vi "conversion_Consigne_UI_Param_FPGA.vi"(10 "customParam":T1={"CamDelayToOpen(µs)"=10, "FLWidth(µs)"=10, "QSWidth(µs)"=10, "DelayFL_QS (µs)"=180, "CamDelayToClose(µs)"=100, "CamPivExposure(µs)"=100}, 11 "Config UI":T3) -> (3 "Config FPGA":T2 {"t_periode" min=1 max=999999 step=1})   [LabVIEW 2023]
uses:
  configUtilisateur.ctl
  configFPGA.ctl
  customParam.ctl
  modeAcq.ctl
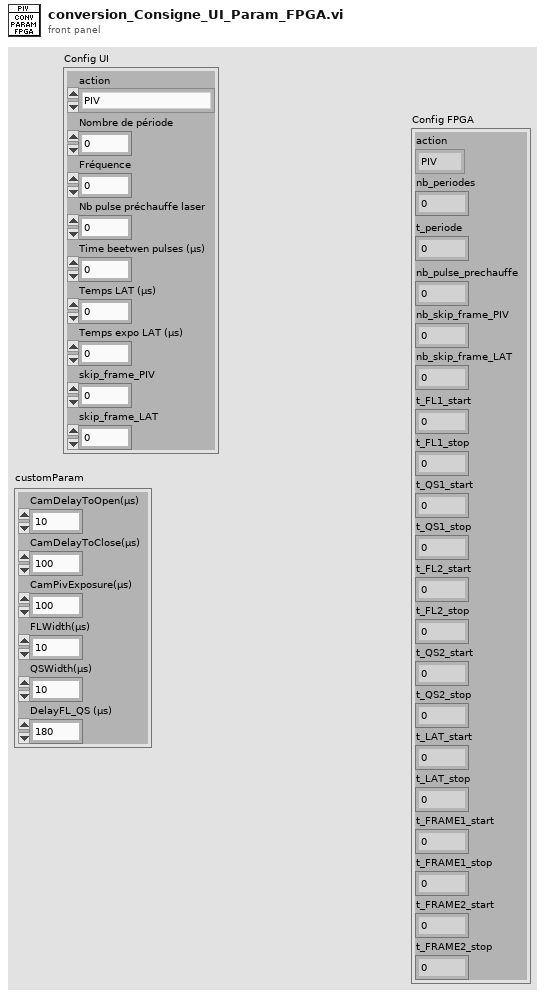
[diagram p1: front panel]
types:
  T1 = typedef "customParam.ctl" = cluster{"CamDelayToOpen(µs)":u32, "FLWidth(µs)":u32, "QSWidth(µs)":u32, "DelayFL_QS (µs)":u32, "CamDelayToClose(µs)":u32, "CamPivExposure(µs)":u32}
  T2 = typedef "configFPGA.ctl" = cluster{"action":enum8{"PIV", "PIV + LAT", "LAT", "STOP"}, "nb_periodes":u16, "t_periode":u32, "nb_pulse_prechauffe":u8, "nb_skip_frame_PIV":u8, "nb_skip_frame_LAT":u8, "t_FL1_start":u32, "t_FL1_stop":u32, "t_QS1_start":u32, "t_QS1_stop":u32, "t_FL2_start":u32, "t_FL2_stop":u32, "t_QS2_start":u32, "t_QS2_stop":u32, "t_LAT_start":u32, "t_LAT_stop":u32, "t_FRAME1_start":u32, "t_FRAME1_stop":u32, "t_FRAME2_start":u32, "t_FRAME2_stop":u32}
  T3 = typedef "configUtilisateur.ctl" = cluster{"Nombre de période":u16, "Fréquence ":u16, "Nb pulse préchauffe laser":u16, "skip_frame_PIV":u8, "skip_frame_LAT":u8, "Time beetwen pulses (µs)":u32, "Temps LAT (µs)":u32, "Temps expo LAT (µs)":u32, "action":enum8{"PIV", "PIV + LAT", "LAT"}}
  T4 = typedef "modeAcq.ctl" = enum8{"PIV", "PIV + LAT", "LAT", "STOP"}
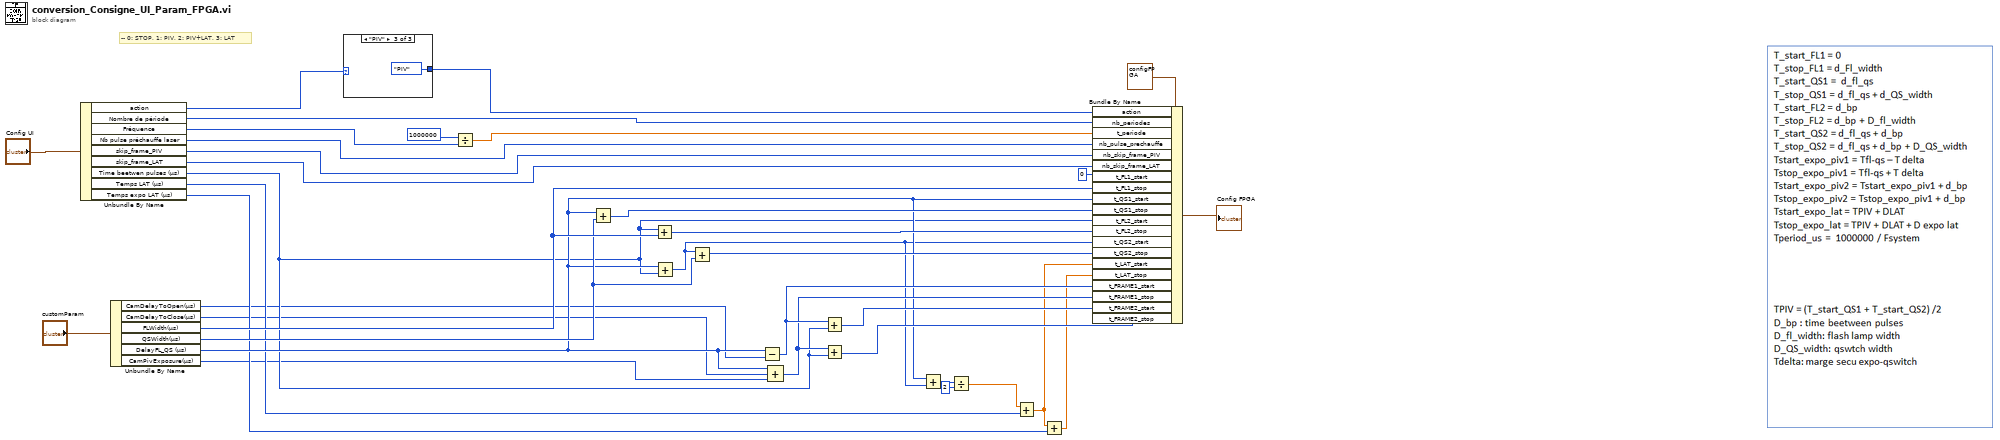
[diagram p0: block diagram]
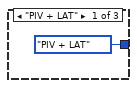
[diagram p2: hidden frame]
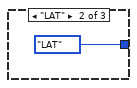
[diagram p3: hidden frame]
diagram:
  # "-- 0: STOP, 1: PIV, 2: PIV+LAT, 3: LAT"
  n1 = Unbundle By Name("Config UI") -> ("action"=w34:enum8{"PIV", "PIV + LAT", "LAT"}, "Nombre de période"=w33:u16, "Fréquence"=w31:u16, "Nb pulse préchauffe laser"=w29:u16, "skip_frame_PIV"=w28:u8, "skip_frame_LAT"=w27:u8, "Time beetwen pulses (µs)"=w12:u32, "Temps LAT (µs)"=w11:u32, "Temps expo LAT (µs)"=w10:u32)
  n2 = Unbundle By Name("customParam") -> ("CamDelayToOpen(µs)"=w4:u32, "CamDelayToClose(µs)"=w3:u32, "FLWidth(µs)"=w23:u32, "QSWidth(µs)"=w21:u32, "DelayFL_QS (µs)"=w16:u32, "CamPivExposure(µs)"=w2:u32)
  n3 = case shown="\"PIV\"" w34 {
    tunnel: [modeAcq."PIV + LAT" ("action") modeAcq."LAT" ("action") modeAcq."PIV" ("action")] -> w1
    frame "PIV + LAT" {
    }
    frame "LAT" {
    }
    frame "PIV" {
    }
  }
  n4 = Divide(x=1000000, y=w31) -> (x/y=w30:dbl)
  n5 = Add(x=w16, y=w21) -> (x+y=w25:u32)
  n6 = Add(x=w12, y=w23) -> (x+y=w24:u32)
  n7 = Add(x=w16, y=w12) -> (x+y=w15:u32)
  n8 = Add(x=w15, y=w21) -> (x+y=w22:u32)
  n9 = Subtract(x=w16, y=w4) -> (x-y=w20:u32)
  n10 = Compound Arithmetic op=ADD(w16, w3, w2) -> (w19:u32)
  n11 = Add(x=w20, y=w12) -> (x+y=w18:u32)
  n12 = Add(x=w19, y=w12) -> (x+y=w17:u32)
  n13 = Add(x=w16, y=w15) -> (x+y=w14:u32)
  n14 = Divide(x=w14, y=u32 2) -> (x/y=w7:dbl)
  n15 = Add(x=w7, y=w11) -> (x+y=w9:dbl)
  n16 = Add(x=w9, y=w10) -> (x+y=w8:dbl)
  n17 = Bundle By Name(cluster=T2 {"action"=enum."PIV + LAT", "nb_periodes"=0, "t_periode"=100000, "nb_pulse_prechauffe"=0, "nb_skip_frame_PIV"=0, "nb_skip_frame_LAT"=0, "t_FL1_start"=0, "t_FL1_stop"=100, "t_QS1_start"=180, "t_QS1_stop"=24, "t_FL2_start"=5000, "t_FL2_stop"=5100, "t_QS2_start"=5180, "t_QS2_stop"=5280, "t_LAT_start"=5680, "t_LAT_stop"=6680, "t_FRAME1_start"=170, "t_FRAME1_stop"=190, "t_FRAME2_start"=5170, "t_FRAME2_stop"=5190} ("Config FPGA"), "action"=w1, "nb_periodes"=w33, "t_periode"=w30, "nb_pulse_prechauffe"=w29, "nb_skip_frame_PIV"=w28, "nb_skip_frame_LAT"=w27, "t_FL1_start"=u32 0, "t_FL1_stop"=w23, "t_QS1_start"=w16, "t_QS1_stop"=w25, "t_FL2_start"=w12, "t_FL2_stop"=w24, "t_QS2_start"=w15, "t_QS2_stop"=w22, "t_LAT_start"=w9, "t_LAT_stop"=w8, "t_FRAME1_start"=w20, "t_FRAME1_stop"=w19, "t_FRAME2_start"=w18, "t_FRAME2_stop"=w17) -> (→"Config FPGA":T2)
